vi "subbus_init.vi"(8 "error in (no error)":errorcluster, 11 "Port":string) -> (0 "error out":errorcluster, 3 "PortOut":string)   [LabVIEW 2016]
uses:
  <vilib>/Instr/_visa.llb/VISA Configure Serial Port (Instr).vi
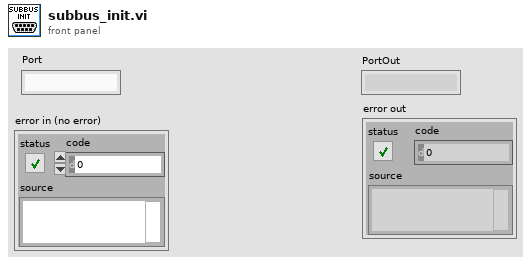
[diagram p1: front panel]
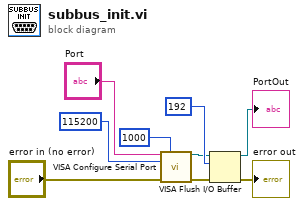
[diagram p0: block diagram]
diagram:
  n1 = call-poly "VISA Configure Serial Port"("VISA resource name"="Port", "timeout (10sec)"=1000, "baud rate (9600)"=115200, "error in (no error)"="error in (no error)") -> ("VISA resource name out"=w5:refnum<visa-resource-name>, "error out"=w4:errorcluster)  [unwired: 10 in]
  n2 = VISA Flush I/O Buffer(VISA resource name=w5, mask (16)=u16 192, error in (no error)=w4) -> (VISA resource name out=→"PortOut":refnum<visa-resource-name>, error out=→"error out":errorcluster)
